vi "Periodic Tasks.vi"(8 "error in":errorcluster) -> ()   [LabVIEW 2017]
doc: "This VI runs in parallel to other robot code. It can contain as many user-defined periodic loops as you need. These can carry out PID or other sorts of timed response."
uses:
  <vilib>/Rock Robotics/SystemInterfaces/spilib/spi_bus.ctl
  <vilib>/Rock Robotics/WPI/Utilities/WPI_GetSetVariantRefNum.vi
  Robot Global Data.vi
  Downloads/ADIS16448-RoboRIO-Driver-master/ADIS16448-RoboRIO-Driver-master/LabVIEW/ADIS16448 IMU/ADIS16448_IMU.lvlib
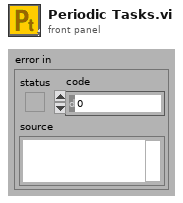
[diagram p1: front panel]
types:
  T1 = typedef "spi_bus.ctl" = enum16{"SPI On-Board, CS0", "SPI On-Board, CS1", "SPI On-Board, CS2", "SPI On-Board, CS3", "SPI MXP", "Invalid"}
  T2 = typedef "ADIS16448_IMU.lvlib/ADI_IMU_ADIS16448_IMUDevRef.ctl" = cluster{"DevStatus":errorcluster, "Handle":i32, "SPI Bus":T1, "Device Found":bool, "Device Ready":bool, "Yaw Axis":enum16{"X", "Y", "Z"}, "AHRS Algorithm":enum16{"Complementary", "Madgwick"}, "Serial":u16, "Lot ID 2":u16, "Lot ID 1":u16, "Bytes Per Sample":u16, "Calibrate On Open?":bool}
  T3 = typedef "WPI_JoystickDevRef.ctl" = cluster{"Device":T4}
  T4 = typedef "WPI_JoystickDeviceEnum.ctl" = enum16{"USB 0", "USB 1", "USB 2", "USB 3", "USB 4", "USB 5"}
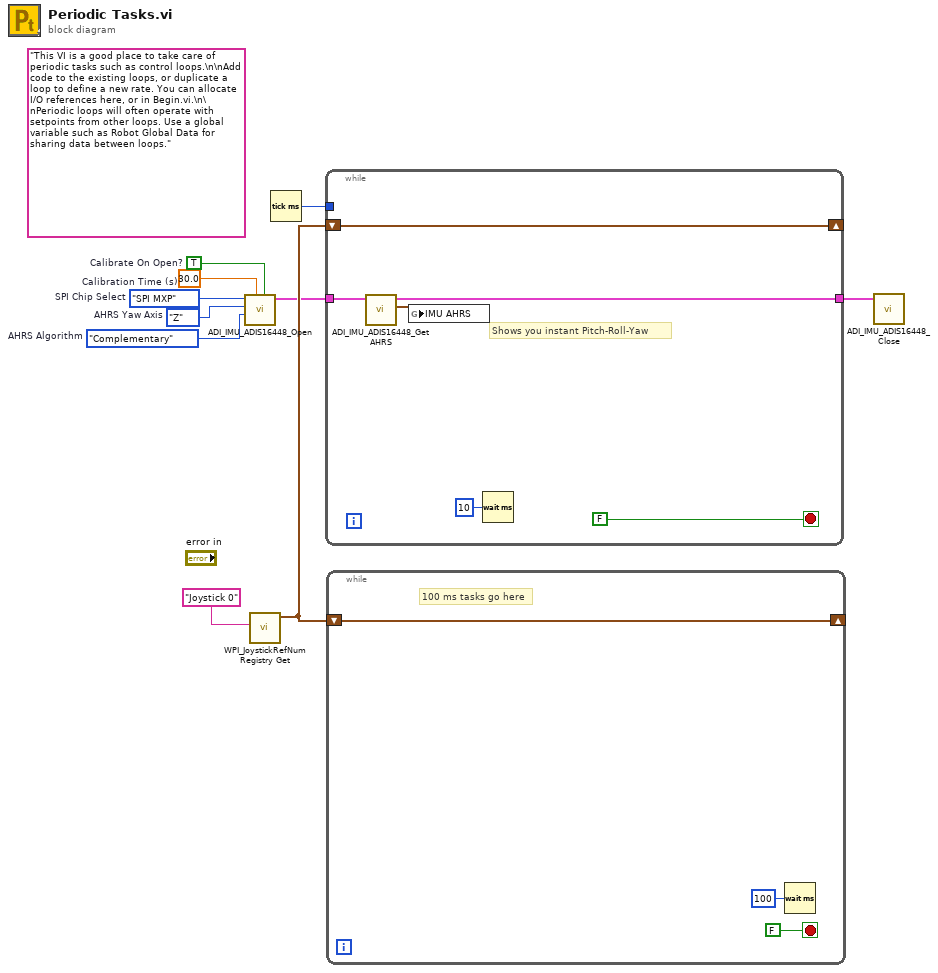
[diagram p0: block diagram]
diagram:
  w7 = enum16{"Complementary", "Madgwick"}."Complementary"  # AHRS Algorithm
  w5 = enum16{"X", "Y", "Z"}."Z"  # AHRS Yaw Axis
  w4 = 30.0  # Calibration Time (s)
  w3 = TRUE  # Calibrate On Open?
  w6 = spi_bus."SPI MXP"  # SPI Chip Select
  (unwired) "This VI is a good place to take care of periodic tasks such as control loops.\n\nAdd code to the existing loops, or duplicate a loop to define a new rate. You can allocate I/O references here, or in Begin.vi.\n\nPeriodic loops will often operate with setpoints from other loops. Use a global variable such as Robot Global Data for sharing data between loops."
  n1 = call "ADI_IMU_ADIS16448_Open.vi"("Calibrate On Open"=w3, "Calibration Time (s)"=w4, "AHRS Algorithm"=w7, "Yaw Axis"=w5, "SPI Chip Select"=w6) -> ("ADI IMU DevRef Out"=w2:T2)  [unwired: 4 in, 2 out]
  n2 = call <vilib>:"WPI_JoystickRefNum Registry Get.vi"("refnum name"="Joystick 0") -> ("JoystickDevRef"=w9:T3)  [unwired: 1 in, 9 out]
  n3 = Tick Count (ms)() -> (millisecond timer value=w8:u32)
  n4 = while {
    shift-right: [w15] -> _
    shift-left: w9 -> [w15]
    tunnel: w8 -> [_]
    tunnel: w2 -> [w13]
    tunnel: [w12] -> w1
    stop <- FALSE stop-if-true
    # "Shows you instant Pitch-Roll-Yaw"
    n5 = call "ADI_IMU_ADIS16448_Get AHRS.vi"("ADI IMU DevRef"=w13) -> ("IMU AHRS Out"=w11:cluster{"Pitch":dbl, "Roll":dbl, "Yaw":dbl}, "ADI IMU DevRef Out"=w12:T2)  [unwired: 7 in, 2 out]
    n6 = global write "Robot Global Data.vi" "IMU AHRS"(w11) -> ()
    n7 = Wait (ms)(milliseconds to wait=u32 10) -> ()  [unwired: 1 out]
  }
  n8 = while {
    shift-right: [w17] -> _
    shift-left: w9 -> [w17]
    stop <- FALSE stop-if-true
    # "100 ms tasks go here"
    n9 = Wait (ms)(milliseconds to wait=u32 100) -> ()  [unwired: 1 out]
  }
  n10 = call "ADI_IMU_ADIS16448_Close.vi"("ADI IMU DevRef"=w1) -> ()  [unwired: 10 in, 1 out]
